vi "niDTS WLAN OFDM Tx Test UTIL WLAN Tx to OFDM Tx Parameters.vi"(7 "WLAN Tx Parameters":T9={"Standard"=enum."802.11 n HT", "DSSS Data Rate (Mbps)"=enum."1", "OFDM Data Rate (Mbps)"=enum."54", "MCS Index"=7, "N spatial streams"=1, "Chains"=[TRUE, FALSE, FALSE, FALSE], "BandWidth (Hz)"=enum."20 MHz", "Channel"=1, "Gard Interval"=enum."SHORT", "FEC Coding"=enum."LDPC", "Dut Tx Power"=0.0, "16 symbols"=TRUE, "payload length bytes"=1500, "idle interval"=0.0001, "External Attenuation"=[0.0, 0.0, 0.0, 0.0], "Acquisition Parameters "={"Acquisition Length Mode"=enum."AUTO", "Acquisition Length (s)"=0.00015, "Auto Level"=FALSE}, "TXP Measurement Parameters"={"TXP Power Enable"=TRUE, "TXP Averages"=3}, "ModAcc Measurement Paramaters"={"ModAcc Enable"=TRUE, "Header Detection"=enum."MANUAL", "Averages"=3, "Amplitude Tracking"=FALSE, "Channel Tracking"=FALSE, "Time Tracking"=TRUE, "Phase Tracking"=enum."NONE", "Clock Offset Est"=FALSE, "Impairments Est"=FALSE, "CFO Estimation"=enum."PAMBLE"}, "ModAcc DSSS Paramaters"={"DC Offset Compensation"=FALSE, "Equalization"=FALSE, "Phase Tracking"=TRUE, "Chip Start Location"=0, "Max Chips Used"=1000, "Pulse Shaping FilterType"=enum."NONE", "Pulse Shaping Filter Coefficient"=0.5}, "SEM Measurement Parameters"={"SEM Enable"=TRUE, "SEM Averages"=3, "Auto Span Enable"=TRUE, "Frequency Span (Hz)"=66000000.0, "Measurement Type"=enum."Standard", "Mask Frequencies (Hz)"=[], "Mask Power Offsets (dB)"=[]}, "OBW Measurement Parameters"={"OBW Enable"=TRUE, "OBW Averages"=3}, "DSSS Power Ramp"={"Power Ramp Enable"=FALSE, "Averages"=3, "Thresholds"={"Up Low (%)"=10.0, "Down Low (%)"=10.0, "Up High (%)"=90.0, "Down High (%)"=90.0}}, "Enable Traces"=FALSE} {"DSSS Power Ramp"."Thresholds"."Down High (%)" min=0.0 max=100.0 step=1.0; "DSSS Power Ramp"."Thresholds"."Up High (%)" min=0.0 max=100.0 step=1.0; "DSSS Power Ramp"."Thresholds"."Down Low (%)" min=0.0 max=100.0 step=1.0; "DSSS Power Ramp"."Thresholds"."Up Low (%)" min=0.0 max=100.0 step=1.0; "Acquisition Parameters"."Acquisition Length (s)" format="%#_6p"; "SEM Measurement Parameters"."Frequency Span (Hz)" format="%#_6p"; "idle interval" format="%_3p"}) -> (8 "OFDM Parameters":T1={"OFDM Data Rate (Mbps)"=enum."54", "Chains"=[TRUE, FALSE, FALSE, FALSE], "Bandwidth (Hz)"=enum."20 MHz", "Channel"=1, "Dut Tx Power (dBm)"=0.0, "16 symbols"=TRUE, "Payload Length (bytes)"=1500, "Idle Interval (s)"=0.0001, "External Attenuation (dB)"=[0.0, 0.0, 0.0, 0.0], "Acquisition "={"Acquisition Length Mode"=enum."AUTO", "Acquisition Length (s)"=3.0, "Auto Level"=FALSE}, "TXP Measurement"={"TXP Power Enable"=FALSE, "TXP Averages"=3}, "ModAcc Measurement"={"ModAcc Enable"=FALSE, "Header Detection"=enum."MANUAL", "Averages"=3, "CFO Estimation"=enum."PAMBLE", "Amplitude Tracking"=FALSE, "Channel Tracking"=FALSE, "Time Tracking"=FALSE, "Phase Tracking"=enum."NONE", "Clock Offset Est"=FALSE, "Impairments Est"=FALSE}, "SEM Measurement"={"SEM Enable"=FALSE, "SEM Averages"=3, "Auto Span Enable"=FALSE, "Frequency Span (Hz)"=0.0, "Measurement Type"=enum."Standard", "Mask Frequencies (Hz)"=[], "Mask Power Offsets (dB)"=[]}, "OBW Measurement"={"OBW Enable"=FALSE, "OBW Averages"=3}} {"Acquisition"."Acquisition Length (s)" format="%#_6p"; "SEM Measurement"."Frequency Span (Hz)" format="%#_6p"; "Idle Interval (s)" format="%_3p"})   [LabVIEW 2014, in "niDTS WLAN.lvlib"]
uses:
  niDTS WLAN.lvlib
  Tx Test/Includes/niDTS WLAN Tx Test INC Parameters.ctl
  Includes/niDTS WLAN INC Standard.ctl
  Includes/niDTS WLAN INC DSSS Data Rate.ctl
  Includes/niDTS WLAN INC OFDM Data Rate.ctl
  Includes/niDTS WLAN INC CH BW.ctl
  Includes/niDTS WLAN INC GI.ctl
  Includes/niDTS WLAN INC FEC Coding.ctl
  Includes/niDTS WLAN DUT INC Acquisition Parameters.ctl
  Includes/niDTS WLAN INC TXP Measurement Parameters.ctl
  Includes/niDTS WLAN INC ModAcc Measurement Parameters.ctl
  Includes/niDTS WLAN INC DSSS ModAcc Measurement Parameters.ctl
  Includes/niDTS WLAN INC Pulse Shaping Filter Type.ctl
  Includes/niDTS WLAN INC SEM Measurement Parameters.ctl
  Includes/niDTS WLAN INC OBW Measurement Parameters.ctl
  Includes/niDTS WLAN INC DSSS Power Ramp Parameters.ctl
  Includes/niDTS WLAN OFDM Tx Test INC Parameters.ctl
  Includes/niDTS WLAN INC CH BW DSSS.ctl
  Includes/niDTS WLAN OFDM Tx Test INC ModAcc Measurement Parameters.ctl
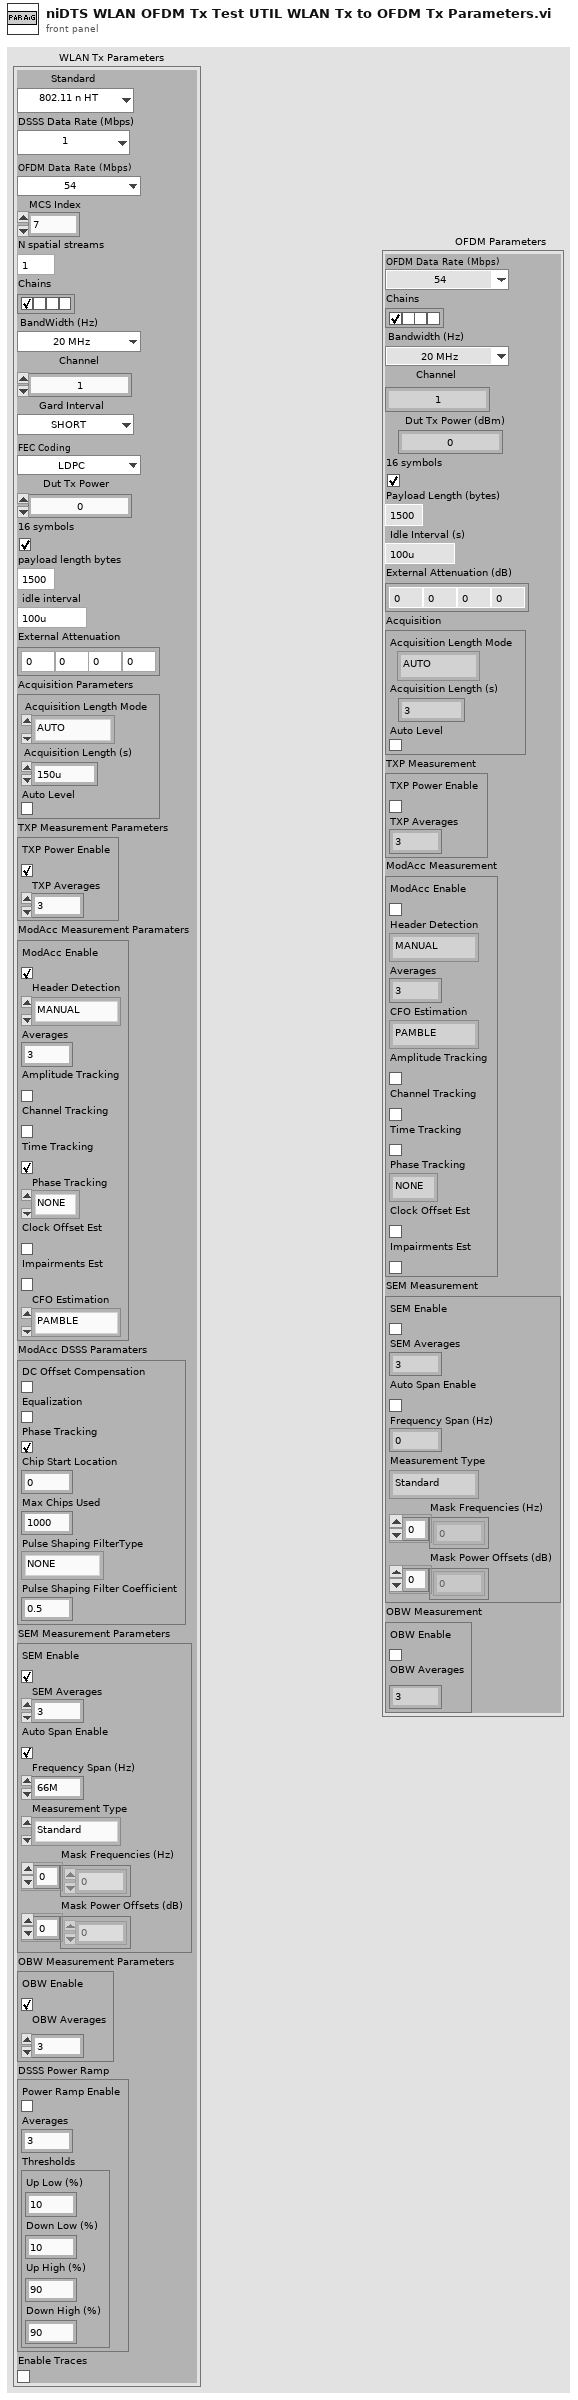
[diagram p1: front panel]
types:
  T1 = typedef "niDTS WLAN.lvlib/niDTS WLAN OFDM Tx Test INC Parameters.ctl" = cluster{"OFDM Data Rate (Mbps)":T2, "Chains":bool[], "Bandwidth (Hz)":T3, "Channel":i32, "Dut Tx Power (dBm)":dbl, "16 symbols":bool, "Payload Length (bytes)":i32, "Idle Interval (s)":dbl, "External Attenuation (dB)":dbl[], "Acquisition ":T4, "TXP Measurement":T5, "ModAcc Measurement":T6, "SEM Measurement":T7, "OBW Measurement":T8}
  T2 = typedef "niDTS WLAN.lvlib/niDTS WLAN INC OFDM Data Rate.ctl" = enum16{"6", "9", "12", "18", "24", "36", "48", "54"}
  T3 = typedef "niDTS WLAN.lvlib/niDTS WLAN INC CH BW DSSS.ctl" = enum16{"20 MHz"}
  T4 = typedef "niDTS WLAN.lvlib/niDTS WLAN DUT INC Acquisition Parameters.ctl" = cluster{"Acquisition Length Mode":enum16{"AUTO", "MANUAL"}, "Acquisition Length (s)":dbl, "Auto Level":bool}
  T5 = typedef "niDTS WLAN.lvlib/niDTS WLAN INC TXP Measurement Parameters.ctl" = cluster{"TXP Power Enable":bool, "TXP Averages":i32}
  T6 = typedef "niDTS WLAN.lvlib/niDTS WLAN OFDM Tx Test INC ModAcc Measurement Parameters.ctl" = cluster{"ModAcc Enable":bool, "Header Detection":enum16{"MANUAL", "FIRST", "ALL"}, "Averages":i32, "CFO Estimation":enum16{"PAMBLE", "PDATA"}, "Amplitude Tracking":bool, "Channel Tracking":bool, "Time Tracking":bool, "Phase Tracking":enum16{"NONE", "STANDARD", "CSF", "INSTANT"}, "Clock Offset Est":bool, "Impairments Est":bool}
  T7 = typedef "niDTS WLAN.lvlib/niDTS WLAN INC SEM Measurement Parameters.ctl" = cluster{"SEM Enable":bool, "SEM Averages":i32, "Auto Span Enable":bool, "Frequency Span (Hz)":dbl, "Measurement Type":enum16{"Standard", "Legacy", "Custom"}, "Mask Frequencies (Hz)":dbl[], "Mask Power Offsets (dB)":dbl[]}
  T8 = typedef "niDTS WLAN.lvlib/niDTS WLAN INC OBW Measurement Parameters.ctl" = cluster{"OBW Enable":bool, "OBW Averages":i32}
  T9 = typedef "niDTS WLAN.lvlib/niDTS WLAN Tx Test INC Parameters.ctl" = cluster{"Standard":T10, "DSSS Data Rate (Mbps)":T11, "OFDM Data Rate (Mbps)":T2, "MCS Index":i32, "N spatial streams":i32, "Chains":bool[], "BandWidth (Hz)":T12, "Channel":i32, "Gard Interval":T13, "FEC Coding":T14, "Dut Tx Power":dbl, "16 symbols":bool, "payload length bytes":i32, "idle interval":dbl, "External Attenuation":dbl[], "Acquisition Parameters ":T4, "TXP Measurement Parameters":T5, "ModAcc Measurement Paramaters":T15, "ModAcc DSSS Paramaters":T16, "SEM Measurement Parameters":T7, "OBW Measurement Parameters":T8, "DSSS Power Ramp":T18, "Enable Traces":bool}
  T10 = typedef "niDTS WLAN.lvlib/niDTS WLAN INC Standard.ctl" = enum16{"802.11 b DSSS", "802.11 a/g OFDM", "802.11 n HT", "802.11 ac VHT"}
  T11 = typedef "niDTS WLAN.lvlib/niDTS WLAN INC DSSS Data Rate.ctl" = enum16{"1", "2", "5.5", "11"}
  T12 = typedef "niDTS WLAN.lvlib/niDTS WLAN INC CH BW.ctl" = enum16{"20 MHz", "40 MHz", "80 MHz", "160 MHz"}
  T13 = typedef "niDTS WLAN.lvlib/niDTS WLAN INC GI.ctl" = enum16{"LONG", "SHORT"}
  T14 = typedef "niDTS WLAN.lvlib/niDTS WLAN INC FEC Coding.ctl" = enum16{"BCC", "LDPC"}
  T15 = typedef "niDTS WLAN.lvlib/niDTS WLAN INC ModAcc Measurement Parameters.ctl" = cluster{"ModAcc Enable":bool, "Header Detection":enum16{"MANUAL", "FIRST", "ALL"}, "Averages":i32, "Amplitude Tracking":bool, "Channel Tracking":bool, "Time Tracking":bool, "Phase Tracking":enum16{"NONE", "STANDARD", "CSF", "INSTANT"}, "Clock Offset Est":bool, "Impairments Est":bool, "CFO Estimation":enum16{"PAMBLE", "PDATA"}}
  T16 = typedef "niDTS WLAN.lvlib/niDTS WLAN INC DSSS ModAcc Measurement Parameters.ctl" = cluster{"DC Offset Compensation":bool, "Equalization":bool, "Phase Tracking":bool, "Chip Start Location":i16, "Max Chips Used":i16, "Pulse Shaping FilterType":T17, "Pulse Shaping Filter Coefficient":dbl}
  T17 = typedef "niDTS WLAN.lvlib/niDTS WLAN INC Pulse Shaping Filter Type.ctl" = enum16{"NONE", "RCOSINE", "RRCOSINE", "GAUSSIAN"}
  T18 = typedef "niDTS WLAN.lvlib/niDTS WLAN INC DSSS Power Ramp Parameters.ctl" = cluster{"Power Ramp Enable":bool, "Averages":i32, "Thresholds":cluster{"Up Low (%)":dbl, "Down Low (%)":dbl, "Up High (%)":dbl, "Down High (%)":dbl}}
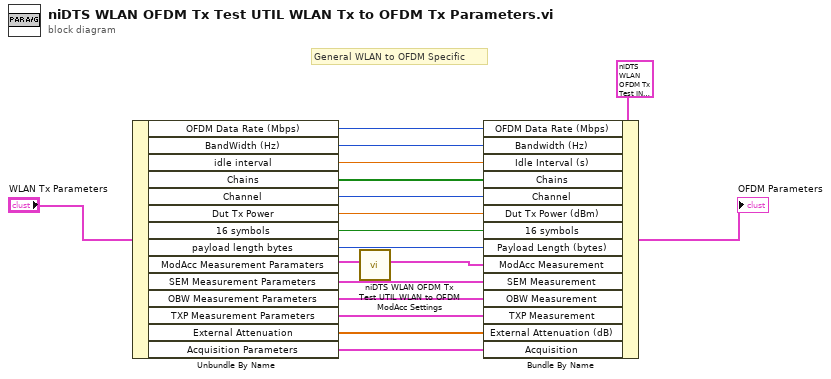
[diagram p0: block diagram]
diagram:
  # "General WLAN to OFDM Specific"
  n1 = Unbundle By Name("WLAN Tx Parameters") -> ("OFDM Data Rate (Mbps)"=w11:T2, "BandWidth (Hz)"=w12:T12, "idle interval"=w13:dbl, "Chains"=w14:bool[], "Channel"=w15:i32, "Dut Tx Power"=w16:dbl, "16 symbols"=w17:bool, "payload length bytes"=w18:i32, "ModAcc Measurement Paramaters"=w9:T15, "SEM Measurement Parameters"=w6:T7, "OBW Measurement Parameters"=w5:T8, "TXP Measurement Parameters"=w4:T5, "External Attenuation"=w3:dbl[], "Acquisition Parameters"=w1:T4)
  n2 = call "niDTS WLAN OFDM Tx Test UTIL WLAN to OFDM ModAcc Settings.vi"("ModAcc Measurement Paramaters"=w9) -> ("OFDM ModAcc Measurement Paramaters"=w7:T6)  [unwired: 10 in]
  n3 = Bundle By Name(cluster=T1 {"OFDM Data Rate (Mbps)"=enum."54", "Chains"=[TRUE, FALSE, FALSE, FALSE], "Bandwidth (Hz)"=enum."20 MHz", "Channel"=1, "Dut Tx Power (dBm)"=0.0, "16 symbols"=TRUE, "Payload Length (bytes)"=1500, "Idle Interval (s)"=0.0001, "External Attenuation (dB)"=[0.0, 0.0, 0.0, 0.0], "Acquisition "={"Acquisition Length Mode"=enum."AUTO", "Acquisition Length (s)"=1.0, "Auto Level"=FALSE}, "TXP Measurement"={"TXP Power Enable"=FALSE, "TXP Averages"=3}, "ModAcc Measurement"={"ModAcc Enable"=FALSE, "Header Detection"=enum."MANUAL", "Averages"=3, "CFO Estimation"=enum."PAMBLE", "Amplitude Tracking"=FALSE, "Channel Tracking"=FALSE, "Time Tracking"=FALSE, "Phase Tracking"=enum."NONE", "Clock Offset Est"=FALSE, "Impairments Est"=FALSE}, "SEM Measurement"={"SEM Enable"=FALSE, "SEM Averages"=3, "Auto Span Enable"=TRUE, "Frequency Span (Hz)"=0.0, "Measurement Type"=enum."Standard", "Mask Frequencies (Hz)"=[], "Mask Power Offsets (dB)"=[]}, "OBW Measurement"={"OBW Enable"=FALSE, "OBW Averages"=3}} ("OFDM Parameters"), "OFDM Data Rate (Mbps)"=w11, "Bandwidth (Hz)"=w12, "Idle Interval (s)"=w13, "Chains"=w14, "Channel"=w15, "Dut Tx Power (dBm)"=w16, "16 symbols"=w17, "Payload Length (bytes)"=w18, "ModAcc Measurement"=w7, "SEM Measurement"=w6, "OBW Measurement"=w5, "TXP Measurement"=w4, "External Attenuation (dB)"=w3, "Acquisition"=w1) -> (→"OFDM Parameters":T1)
